vi "Board Tick.vi"(8 "error in (no error)":errorcluster, 11 "Board in":refnum<class "Board.lvclass">) -> (0 "error out":errorcluster, 1 "Score Updates":refnum<class "Player.lvclass">[](array[class]), 2 "Dead Players":refnum<class "Player.lvclass">[](array[class]), 3 "Board out":refnum<class "Board.lvclass">)   [LabVIEW 2019, in "Board.lvclass"]
uses:
  Board.lvclass
  Board.lvclass/Board.ctl
  Player/Player.lvclass
  Food/Food.lvclass
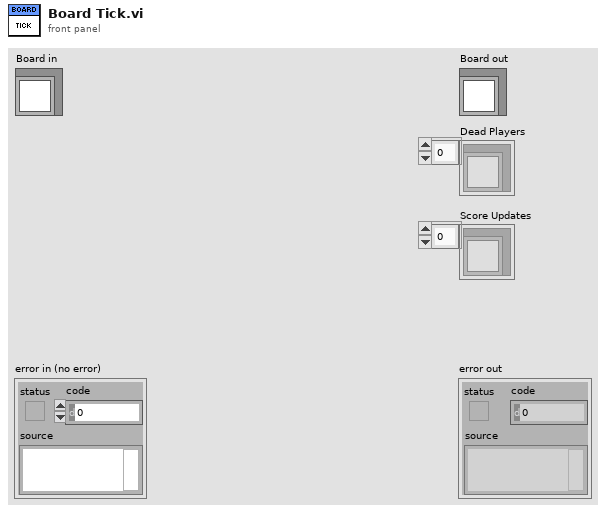
[diagram p1: front panel]
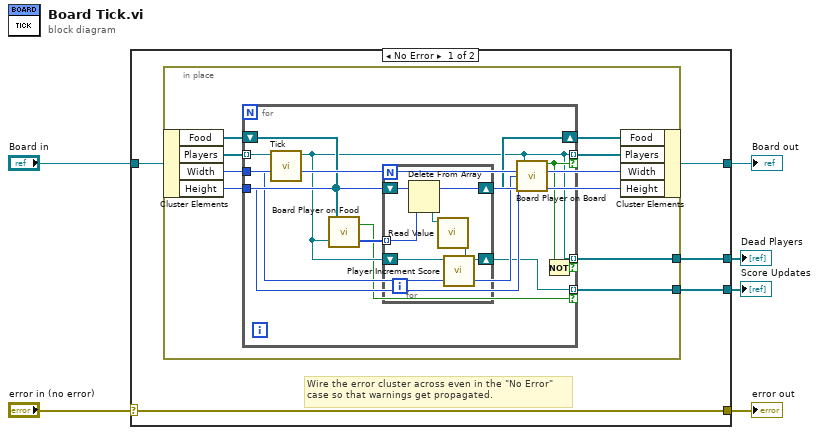
[diagram p0: block diagram]
diagram:
  n1 = case shown="No Error" "error in (no error)" {
    selector: "error in (no error)" -> [w11 w39]
    tunnel: [w11 w39] -> w5
    tunnel: [w10 w38] -> w3
    tunnel: "Board in" -> [w9 w38]
    tunnel: [w8 _] -> w2
    tunnel: [w7 _] -> w1
    frame No Error {
      # "Wire the error cluster across even in the \"No Error\"\ncase so that warnings get propagated."
      n2 = in-place {
        in-place-border: [w13] -> w8
        in-place-border: [w12] -> w7
        n3 = in-place-cluster #1(w9) -> ("Food"=w19:refnum<class "Food.lvclass">[], "Players"=w18:refnum<class "Player.lvclass">[], "Width"=w15:i32, "Height"=w14:i32)
        n4 = for {
          tunnel: w18 -> [w30] mode=indexing
          shift-right: [w27] -> w17
          shift-left: w19 -> [w28]
          tunnel: [w22] -> w16 mode=indexing if=w24
          tunnel: w15 -> [w26]
          tunnel: w14 -> [w25]
          tunnel: [w22] -> w13 mode=indexing if=w23
          tunnel: [w21] -> w12 mode=indexing if=w20
          n5 = call-dynamic "Tick.vi"("Player in"=w30) -> ("Player out"=w22:refnum<class "Player.lvclass">)  [unwired: 9 in, 1 out]
          n6 = call "Board Player on Food.vi"("Player"=w22, "Food"=w28) -> ("Indices"=w29:i32[], "Found?"=w20:bool)
          n7 = for {
            tunnel: w29 -> [w35] mode=indexing
            shift-right: [w36] -> w27
            shift-left: w28 -> [w37]
            shift-right: [w31] -> w21
            shift-left: w22 -> [w33]
            n8 = Delete From Array(array=w37, index=w35) -> (deleted portion=w34:refnum<class "Food.lvclass">, array with subset deleted=w36:refnum<class "Food.lvclass">[])  [unwired: 1 in]
            n9 = call-dynamic "Read Value.vi"("Food in"=w34) -> ("Value"=w32:i32)  [unwired: 8 in, 2 out]
            n10 = call-dynamic "Player Increment Score.vi"("Amount"=w32, "Player in"=w33) -> ("Player out"=w31:refnum<class "Player.lvclass">)  [unwired: 8 in, 1 out]
          }
          n11 = call "Board Player on Board.vi"("Height"=w25, "Width"=w26, "Player"=w22) -> ("In Range?"=w24:bool)
          n12 = Not(x=w24) -> (.not. x?=w23:bool)
        }
        n13 = in-place-cluster #1("Food"=w17, "Players"=w16, "Width"=w15, "Height"=w14) -> (w10:refnum<class "Board.lvclass">)
      }
    }
    frame Error {
    }
  }
  "error out" <- w5
  "Board out" <- w3
  "Dead Players" <- w2
  "Score Updates" <- w1
